vi "Thread@ErrorRetry__Parameter.vi"(1 "ParamterIn":string) -> (0 "ParamterOut":string)   [LabVIEW 2020]
panel:
  in  "Offset":string(combo)
  in  "Logic":string(combo)
  in  "Confirm":bool
  # "Thread@ErrorRetry ($Logic,$ReturnOffset)"
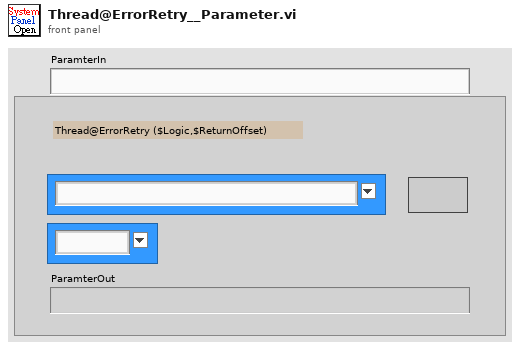
[diagram p1: front panel]
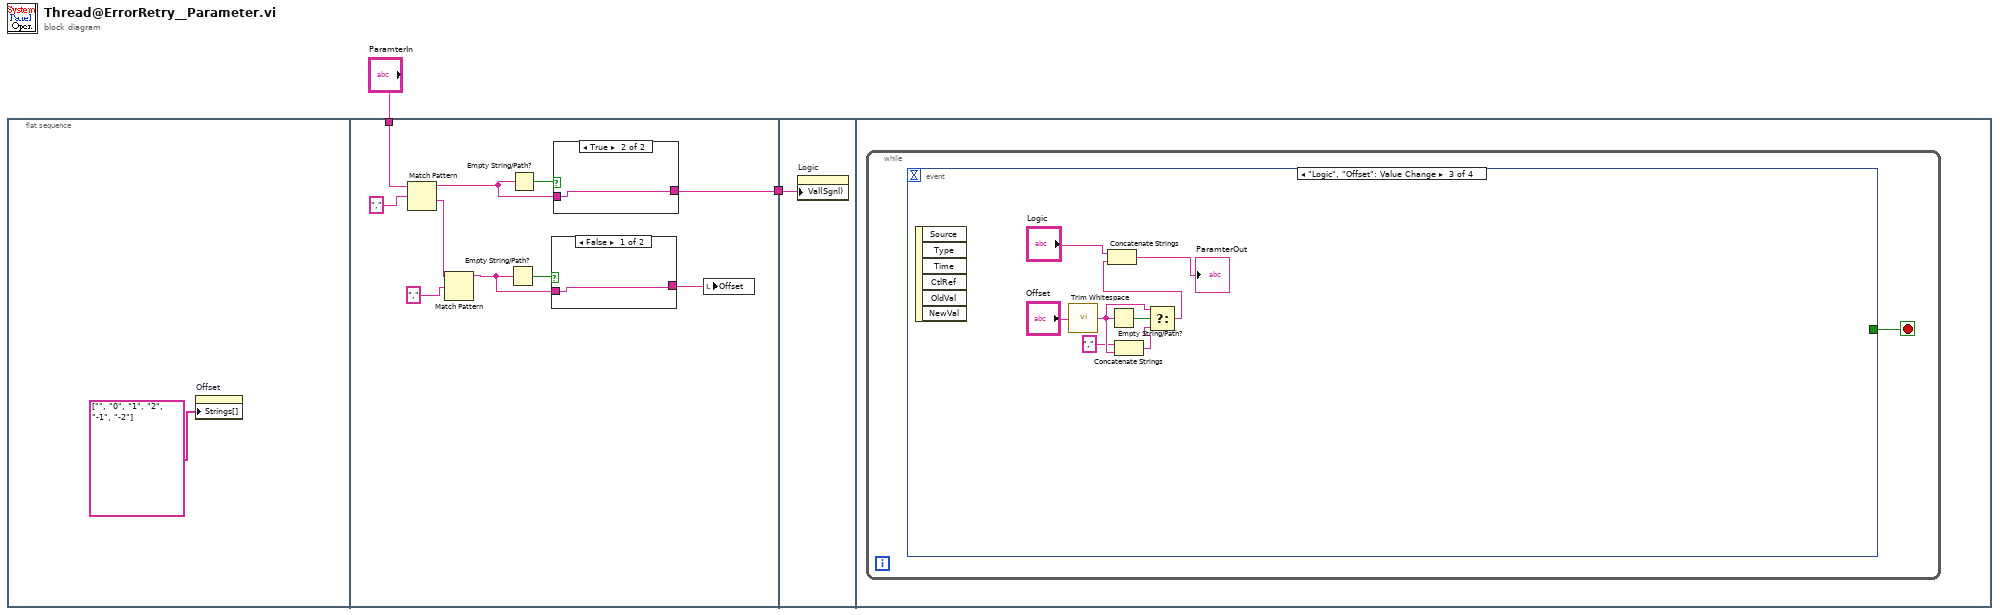
[diagram p0: block diagram]
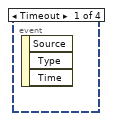
[diagram p4: hidden frame]
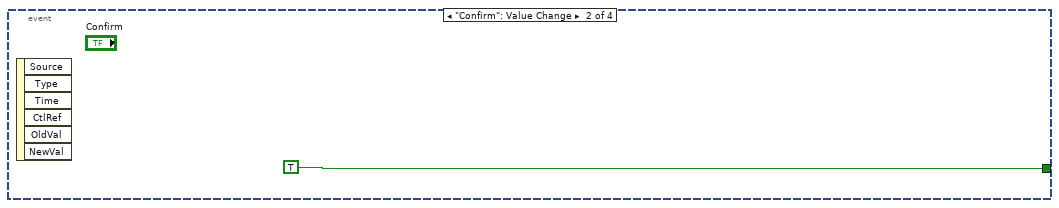
[diagram p5: hidden frame]
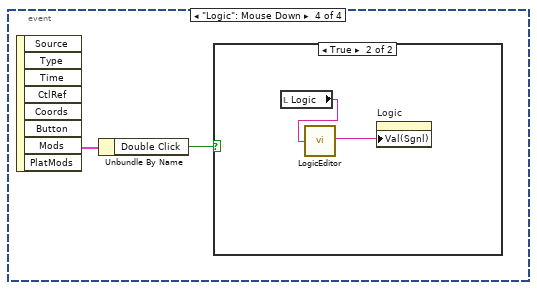
[diagram p6: hidden frame]
diagram:
  n1 = flat-sequence {
    tunnel: "ParamterIn" -> [w12]
    tunnel: [w8] -> w1
    tunnel: w1 -> [w18]
    frame #0 {
      n2 = property on="Offset" class="CmbBox"("Strings[]"=string[] ["", "0", "1", "2", "-1", "-2"] ("Strings []")) -> ()  [unwired: 2 in, 2 out]
    }
    frame #1 {
      n3 = Match Pattern(string=w12, regular expression=",") -> (before substring=w10:string, after substring=w5:string)  [unwired: 1 in, 2 out]
      n4 = Match Pattern(string=w5, regular expression=",") -> (before substring=w4:string)  [unwired: 1 in, 3 out]
      n5 = Empty String/Path?(string/path=w4) -> (empty?=w9:bool)
      n6 = Empty String/Path?(string/path=w10) -> (empty?=w13:bool)
      n7 = case shown="False" w9 {
        tunnel: w4 -> [w14 w15]
        tunnel: [w14 w15] -> w7
        frame False {
        }
        frame True {
        }
      }
      n8 = case shown="True" w13 {
        tunnel: w10 -> [w16 w17]
        tunnel: [w16 w17] -> w8
        frame False {
        }
        frame True {
        }
      }
      n9 = local write "Offset"(w7) -> ()
    }
    frame #2 {
      n10 = property on="Logic" class="CmbBox"("Val(Sgnl)"=w18) -> ()  [unwired: 2 in, 2 out]
    }
    frame #3 {
      n11 = while {
        stop <- w19 stop-if-true
        n12 = event shown="[2] \"Logic\", \"Offset\": Value Change" {
          selector: _ -> [_ _ _ _]
          dyn-events: _ -> [_ _ _ _]
          timeout: _ -> [_ _ _ _]
          tunnel: [_ TRUE _ _] -> w19
          event Timeout {
            n13 = event-data() -> ()  [unwired: 1 in, 3 out]
          }
          event "Confirm": Value Change {
            n14 = event-data() -> ()  [unwired: 1 in, 6 out]
          }
          event "Logic", "Offset": Value Change {
            n15 = event-data() -> ()  [unwired: 1 in, 6 out]
            n16 = call <vilib>:"Trim Whitespace.vi"("string"="Offset") -> ("trimmed string"=w23:string)  [unwired: 1 in]
            n17 = Empty String/Path?(string/path=w23) -> (empty?=w25:bool)
            n18 = Concatenate Strings("," ("string"), w23) -> (w24:string)
            n19 = Select(t=w23, s=w25, f=w24) -> (s? t:f=w21:string)
            n20 = Concatenate Strings("Logic", w21) -> (→"ParamterOut":string)
          }
          event "Logic": Mouse Down {
            n21 = event-data() -> ("Mods"=w30:cluster{"Double Click":bool, "Menu Key":bool})  [unwired: 1 in, 7 out]
            n22 = Unbundle By Name(w30) -> ("Double Click"=w29:bool)
            n23 = case shown="True" w29 {
              frame False {
              }
              frame True {
                n24 = local read "Logic"() -> (w32:string)
                n25 = call "LogicEditor.vi"("Logic Express"=w32) -> ("LogicExpressOut"=w31:string)
                n26 = property on="Logic" class="CmbBox"("Val(Sgnl)"=w31) -> ()  [unwired: 2 in, 2 out]
              }
            }
          }
        }
      }
    }
  }
